vi "Climb Loop.vi"() -> ()   [LabVIEW 2015]
uses:
  Robot Global Data.vi
  <vilib>/Rock Robotics/WPI/Solenoid/WPI_SolenoidSetEnum.vi
panel:
  in  "Climb Start":dbl
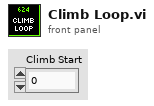
[diagram p1: front panel]
types:
  T1 = typedef "Dashboard Control Data.ctl" = cluster{"Encoder Control":T2, "Steer PID output":cluster{"output high":dbl, "output low":dbl}, " Steer PID gains":cluster{"proportional gain (Kc)":dbl, "integral time (Ti, min)":dbl, "derivative time (Td, min)":dbl}, "Drivetrain Settings":T3, "Vision Packet":T4, "Dashboard Drivetrain Command":T5, "Info/Command Cluster":T7, "Ball Vision Packet":T8, "Intake Presets":T10, "Intake Encoder Control":T12, "Goal Output Range":cluster{"output high":dbl, "output low":dbl}, "Enabled Systems":T13, "Auton Presets":T14, "Pressure M":dbl, "Pressure B":dbl, "Vision Timeout":dbl, "Auto-Shift":T15, "Catapult Setpoints":T16, "Climb Presets":T17}
  T2 = typedef "Encoder Control.ctl" = cluster{"Right Tick Constant":dbl, "Left Tick Constant":dbl, "Reset?":bool, "Y Dist":cluster{"PID gains":cluster{"proportional gain (Kc)":dbl, "integral time (Ti, min)":dbl, "derivative time (Td, min)":dbl}}, "Y Stop Thresh":dbl, "Y Stop Speed":dbl}
  T3 = typedef "Drivetrain Settings.ctl" = cluster{"Gyro Tolerance":dbl, "Throttle Ramp (ms)":dbl, "Kv":dbl, "Ka":dbl, "Feed Forward P":dbl, "Feed Forward D":dbl, "Goal Vision PID gains":cluster{"proportional gain (Kc)":dbl, "integral time (Ti, min)":dbl, "derivative time (Td, min)":dbl}, "Goal Detection Window":dbl, "Creep Rate":dbl, "Vision Throttle Threshold":dbl, "Min Turn Output":dbl, "Left Batter Angle":dbl, "Right Batter Angle":dbl}
  T4 = typedef "Goal Vision Packet.ctl" = cluster{"Distance":dbl, "Center X":dbl, "Center Y":dbl, "Found Target?":bool, "Robot Center":dbl, "Angle":dbl}
  T5 = typedef "Dashboard Drivetrain Command.ctl" = cluster{"Drivetrain Vision":T6}
  T6 = typedef "Drivetrain Vision.ctl" = cluster{"Goal Window":dbl, "Ball Window":dbl}
  T7 = typedef "Ball Tracking Command Cluster.ctl" = cluster{"Distance to Ball":dbl, "Desired Angle":dbl, "Command":enum16{"Turn to Ball", "Turn to Angle", "Get Distance"}, "Pixels from Center":dbl}
  T8 = typedef "Ball Vision Packet.ctl" = cluster{"Ball Detected?":bool, "Distance to Ball":dbl, "Desired Angle":dbl, "Pixels from Center":dbl, "Tracking mode":T9}
  T9 = typedef "Tracking Mode.ctl" = enum16{"Turn to Ball", "Turn to Angle"}
  T10 = typedef "Intake Presets.ctl" = cluster{"Intake Speed":dbl, "Outake Speed":dbl, "Angle Speed":dbl, "Angle Tolerance":dbl, "Encoder Scale":dbl, "Load Height":dbl, "Output Range":T11, "MaxCurrent":dbl, "Idle Height":dbl, "Max Height":dbl, "Reset Encoders?":bool, "PID gains":cluster{"proportional gain (Kc)":dbl, "integral time (Ti, min)":dbl, "derivative time (Td, min)":dbl}, "Drop Low Height ":dbl, "Rotation Power Max/Min":dbl, "Reset Delay":dbl}
  T11 = typedef "Drivetrain Output Range.ctl" = cluster{"output high":dbl, "output low":dbl}
  T12 = typedef "IntakeEcoderControl.ctl" = cluster{"Arm Tick Constant":dbl, "Reset?":bool, "Y Dist":cluster{"PID gains":cluster{"proportional gain (Kc)":dbl, "integral time (Ti, min)":dbl, "derivative time (Td, min)":dbl}}, "Y Stop Thresh":dbl, "Y Stop Speed":dbl}
  T13 = typedef "Enabled Systems.ctl" = cluster{"Shoot":bool, "Intake":bool, "DT":bool, "Gyro":bool, "100ms":bool, "US":bool}
  T14 = typedef "Autonomous Presets.ctl" = cluster{"Pitch Limit":dbl, "Roll Limit":dbl, "Start Position":dbl, "Cross Position":dbl}
  T15 = typedef "Auto Shift Cluster.ctl" = cluster{"Delay":dbl, "Speed Thresh":dbl, "Upshift Accel":dbl, "Upshift Throttle":dbl, "Upshift Throttle Accel":dbl, "Downshift Throttle":dbl, "Downshift Throttle Accel":dbl, "Pressure Threshold":dbl}
  T16 = typedef "Catapult Presets.ctl" = cluster{"Intake Danger Height":dbl, "Ball Security Delay ":dbl, "High PSI Minimum":dbl, "Shot Finish Delay":dbl, "Low PSI Minimum":dbl, "Idle Ball Security Wait ":dbl}
  T17 = typedef "Climb Presets.ctl" = cluster{"Winch Speed":dbl}
  T18 = typedef "WPI_SolenoidDevRef.ctl" = cluster{"DevStatus":errorcluster, "Pneumatics Control Module":u8, "Forward Solenoid Channel":T19, "Reverse Solenoid Channel":T19}
  T19 = typedef "WPI_SolenoidChannel.ctl" = enum8{"Solenoid 0", "Solenoid 1", "Solenoid 2", "Solenoid 3", "Solenoid 4", "Solenoid 5", "Solenoid 6", "Solenoid 7", "Invalid"}
  T20 = typedef "WPI_MotorControlDeviceRef.ctl" = cluster{"DeviceStatus":errorcluster, "Type":T21, "PWM":cluster{"PWM Channel":T22, "DeadBand":T23}, "CAN":cluster{"Device Number":u8, "Control Mode":T24, "Semaphore":T25, "Max Vout":dbl, "TalonSRX Control Mode":T26}, "Invert":bool}
  T21 = typedef "WPI_MotorControlType.ctl" = enum16{"PWM", "CAN", "CANTalonSRX"}
  T22 = typedef "FPGA_DIOPWMChannel.ctl" = enum8{"PWM 0", "PWM 1", "PWM 2", "PWM 3", "PWM 4", "PWM 5", "PWM 6", "PWM 7", "PWM 8", "PWM 9", "PWM MXP 0", "PWM MXP 1", "PWM MXP 2", "PWM MXP 3", "PWM MXP 4", "PWM MXP 5", "PWM MXP 6", "PWM MXP 7", "PWM MXP 8", "PWM MXP 9", "Invalid"}
  T23 = typedef "WPI_PWMDeadband.ctl" = cluster{"Name":string, "maxPositivePwm":i32, "minPositivePwm":i32, "centerPwm":i32, "maxNegativePwm":i32, "minNegativePwm":i32, "angularRange":u16}
  T24 = typedef "WPI_CANJaguar_ControlMode.ctl" = enum8{"Percent VBus", "Current", "Speed", "Position", "Voltage"}
  T25 = typedef "Semaphore RefNum" = refnum<k1>
  T26 = typedef "WPI_CANTalonSRX_APIControlMode.ctl" = enum8{"Percent VBus", "Speed", "Position", "Slave", "Unchanged / Invalid", "Voltage Compensation", "Current", "Motion Profile"}
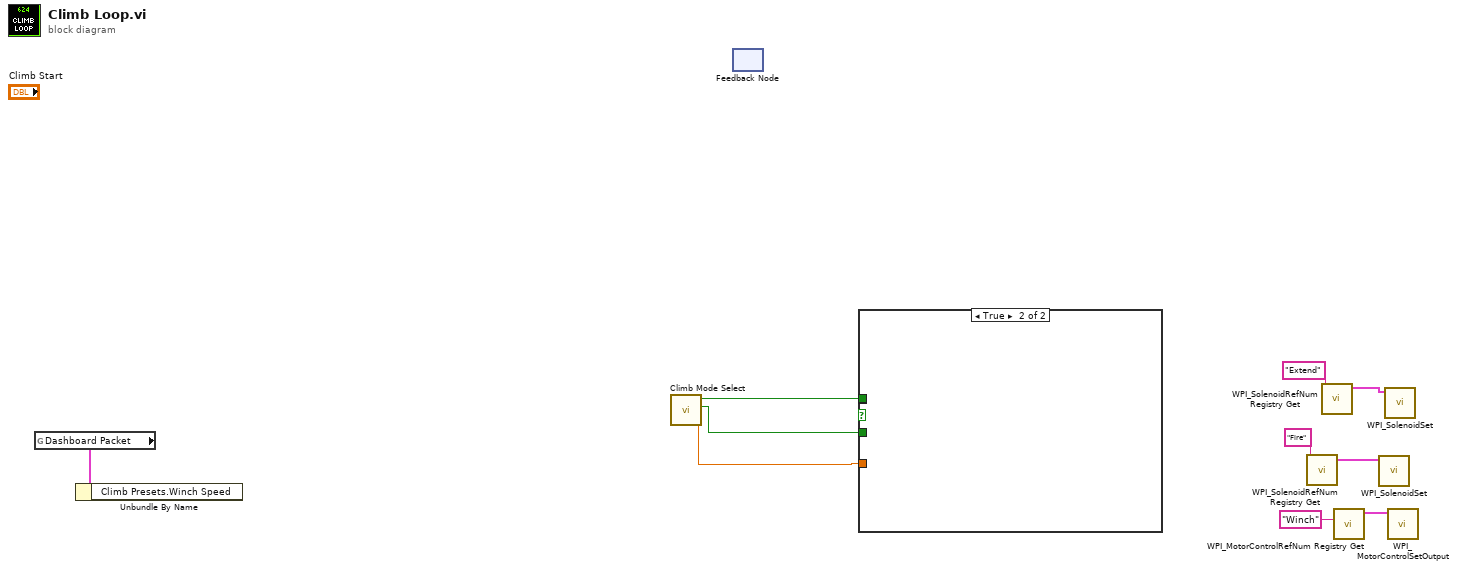
[diagram p0: block diagram]
diagram:
  n1 = global read "Robot Global Data.vi" "Dashboard Packet"() -> (w4:T1)
  n2 = Unbundle By Name(w4) -> ()  [unwired: 1 out]
  n3 = call "Climb Mode Select.vi"() -> ("Winch"=w1:dbl, "Fire?"=w2:bool, "Extend?"=w3:bool)  [unwired: 8 in, 1 out]
  n4 = feedback-in #1() -> ()  [unwired: 1 out]
  n5 = feedback #1() -> ()  [unwired: 2 in]
  n6 = case shown="True" {
    selector: _ -> [_ _]
    tunnel: [w11 _] -> _
    tunnel: w3 -> [w11 _]
    tunnel: w2 -> [_ _]
    tunnel: w1 -> [_ _]
    frame False {
    }
    frame True {
    }
  }
  n7 = call <vilib>:"WPI_SolenoidRefNum Registry Get.vi"("refnum name"="Fire") -> ("SolenoidDevRef"=w6:T18)  [unwired: 9 in, 1 out]
  n8 = call <vilib>:"WPI_SolenoidRefNum Registry Get.vi"("refnum name"="Extend") -> ("SolenoidDevRef"=w5:T18)  [unwired: 9 in, 1 out]
  n9 = call <vilib>:"WPI_MotorControlRefNum Registry Get.vi"("refnum name"="Winch") -> ("MotorControlDevRef"=w9:T20)  [unwired: 9 in, 1 out]
  n10 = call-poly <vilib>:"WPI_SolenoidSet.vi"("SolenoidDevRef"=w6) -> ()  [unwired: 9 in, 2 out]
  n11 = call-poly <vilib>:"WPI_SolenoidSet.vi"("SolenoidDevRef"=w5) -> ()  [unwired: 9 in, 2 out]
  n12 = call <vilib>:"WPI_MotorControlSetOutput.vi"("MotorControlDevRef"=w9) -> ()  [unwired: 8 in, 3 out]
